vi "flush ZMQ standalone.vi"(8 "error in":errorcluster, 9 "Boolean":bool=TRUE, 11 "port":string) -> (0 "error out":errorcluster, 3 "Messages":string[](array[string]))   [LabVIEW 2018]
uses:
  <vilib>/addons/zeromq/zmq_context.lvclass
  <vilib>/addons/zeromq/socket_type.ctl
  <vilib>/addons/zeromq/zeromq.lvlib
  <vilib>/addons/zeromq/zmq_socket.lvclass
  labviewtoolbox/Release 19/StdOut Operations/_subVIs/Append String to StdOut.vi
panel:
  out "Boolean":bool=TRUE
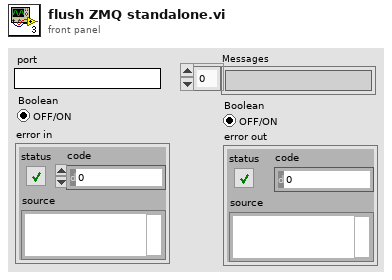
[diagram p1: front panel]
types:
  T1 = typedef "zeromq.lvlib/socket_type.ctl" = enum8{"ZMQ_PAIR", "ZMQ_PUB", "ZMQ_SUB", "ZMQ_REQ", "ZMQ_REP", "ZMQ_DEALER", "ZMQ_ROUTER", "ZMQ_PULL", "ZMQ_PUSH", "ZMQ_XPUB", "ZMQ_XSUB"}
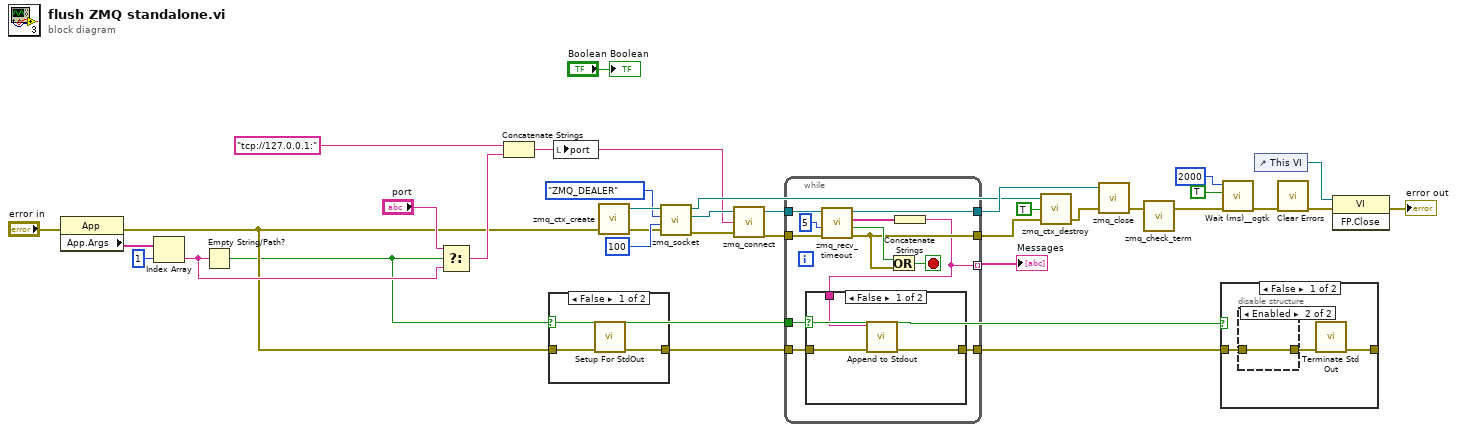
[diagram p0: block diagram]
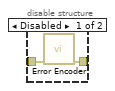
[diagram p2: hidden frame]
diagram:
  n1 = property class="App"(error in="error in") -> (error out=w4:errorcluster, "App.Args"=w14:string[])  [unwired: 1 in, 1 out]
  n2 = Index Array(array=w14, index=1) -> (element=w12:string)
  n3 = Empty String/Path?(string/path=w12) -> (empty?=w1:bool)
  n4 = Select(t="port", s=w1, f=w12) -> (s? t:f=w6:string)
  n5 = Concatenate Strings("tcp://127.0.0.1:" ("ZMQ endpoint 2"), w6) -> (w7:string)
  n6 = case shown="False" w1 {
    tunnel: w4 -> [w37 w38]
    tunnel: [w36 w38] -> w3
    frame False {
      n7 = call "Setup For StdOut.vi"("error in (no error)"=w37) -> ("error out"=w36:errorcluster)  [unwired: 6 in]
    }
    frame True {
    }
  }
  n8 = local write "port"(w7) -> ()
  n9 = call <vilib>:"zmq_ctx_create.vi"("error in"=w4) -> ("error out"=w26:errorcluster, "context out"=w27:refnum<class "zmq_context.lvclass">)  [unwired: 3 in]
  n10 = call <vilib>:"zmq_socket.vi"("error in"=w26, "linger (ms)"=100, "socket type"=socket_type."ZMQ_DEALER", "context in"=w27) -> ("error out"=w25:errorcluster, "socket out"=w24:refnum<class "zmq_socket.lvclass">, "context out"=w31:refnum<class "zmq_context.lvclass">)  [unwired: 1 in]
  n11 = call <vilib>:"zmq_connect.vi"("error in"=w25, "endpoint"=w7, "socket in"=w24) -> ("error out"=w33:errorcluster, "socket out"=w30:refnum<class "zmq_socket.lvclass">)  [unwired: 1 in]
  n12 = while {
    tunnel: w30 -> [w50]
    tunnel: [w44] -> w34
    tunnel: [w41] -> w35 mode=indexing
    tunnel: [w48] -> w32
    tunnel: w33 -> [w47]
    tunnel: w3 -> [w42]
    tunnel: [w40] -> w2
    tunnel: w1 -> [w39]
    stop <- w43 stop-if-true
    n13 = call <vilib>:"zmq_recv_timeout.vi"("error in"=w47, "timeout (ms)"=u32 5, "socket in"=w50) -> ("error out"=w44:errorcluster, "timeout?"=w45:bool, "parts"=w49:string[], "socket out"=w48:refnum<class "zmq_socket.lvclass">)  [unwired: 1 in]
    n14 = Or(x=w45, y=w44) -> (x .or. y?=w43:bool)
    n15 = Concatenate Strings(w49) -> (w41:string)
    n16 = case shown="False" w39 {
      tunnel: w42 -> [w53 w54]
      tunnel: w41 -> [w52 _]
      tunnel: [w51 w54] -> w40
      frame False {
        n17 = call-poly "Append to Stdout.vi"("error in (no error)"=w53, "text"=w52) -> ("error out"=w51:errorcluster)  [unwired: 5 in]
      }
      frame True {
      }
    }
  }
  "Messages" <- w35
  n18 = call <vilib>:"zmq_ctx_destroy.vi"("error in"=w34, "reap? (F)"=TRUE, "context in"=w31) -> ("error out"=w21:errorcluster)  [unwired: 2 in]
  n19 = call <vilib>:"zmq_close.vi"("error in"=w21, "socket"=w32) -> ("error out"=w20:errorcluster)  [unwired: 3 in]
  n20 = call <vilib>:"zmq_check_term.vi"("error in"=w20) -> ("error out"=w11:errorcluster)  [unwired: 1 in, 1 out]
  n21 = case shown="False" w1 {
    tunnel: w2 -> [w57 _]
    tunnel: [w55 _] -> _
    frame False {
      n22 = disable-structure shown="Enabled" {
        disable-tunnel: w57 -> [w59 w60]
        disable-tunnel: [w58 w60] -> w56
        frame Disabled {
          n23 = call "Error Encoder.vi"("error in (no error)"=w59) -> ("error out"=w58:errorcluster)  [unwired: 6 in]
        }
        frame Enabled {
        }
      }
      n24 = call "Terminate Std Out.vi"("error in (no error)"=w56) -> ("error out"=w55:errorcluster)  [unwired: 6 in]
    }
    frame True {
    }
  }
  n25 = call <userlib>:"Wait (ms)__ogtk.vi"("error in (no error)"=w11, "Wait on Error (FALSE)"=TRUE, "milliseconds to wait"=u32 2000) -> ("error out"=w10:errorcluster)  [unwired: 7 in, 1 out]
  n26 = control-ref of="This VI"() -> (w16:refnum<vi>)
  n27 = call <vilib>:"Clear Errors.vi"("error in (no error)"=w10) -> ("error out"=w18:errorcluster)  [unwired: 5 in, 1 out]
  n28 = invoke class="VI" method="FP.Close"(reference=w16, error in=w18) -> (error out=→"error out":errorcluster)  [unwired: 1 in, 2 out]
  "Boolean" <- "Boolean"
